vi "next chunk - read freq PID file.vi"(6 "temperature":dbl, 11 "peaks are known -- parameters":T1={"Gamma (kHz)"=0.0, "dV"=0.0, "time in Gamma (sec)"=0.0, "phi-star"=0.0, "all peaks exp (kHz)"=[564, 649, 987, 1133, 1214, 1585, 1763, 1823, 1880, 1899, 2032, 2138, 2221, 2270, 2350, 2456, 2580, 2634, 2831, 2960, 2965, 3131, 3328, 3469, 3553, 0, 3615, 3734, 0, 0, 0, 4236, 4300, 4331], "delta t (sec)"=0.0, "freq PID file path"=path "E:/data/Ultrasound/Experiment/ProbeTest/Probe10/YBCO_5/sweep4/9w/rus_scan_freq_list.dat", "default step (Hz)"=0.0}) -> (0 "temperatures":i32[](array[numeric]), 1 "frequencies":dbl[][](array[numeric]), 2 "PID freq":dbl[](array[numeric]))   [LabVIEW 2010]
uses:
  next chunk -- parameters.ctl
  <vilib>/Utility/file.llb/Read From Spreadsheet File (string).vi
panel:
  out "number 2":i32=9
  out "number":i32=9
  out "first line":string="Temperature(K)\tFrequency(kHz)\tGamma(kHz)\tDeltaFreq(kHz)\tTime(min)"
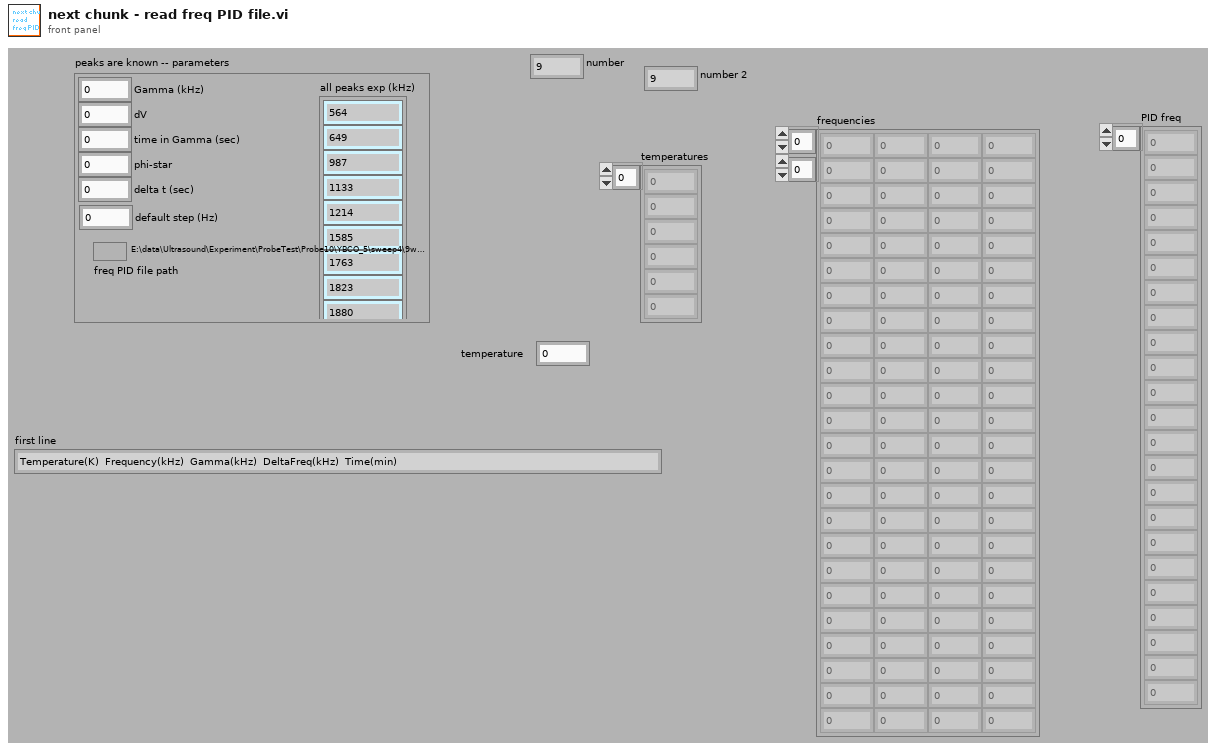
[diagram p1: front panel]
types:
  T1 = typedef "next chunk -- parameters.ctl" = cluster{"Gamma (kHz)":dbl, "dV":dbl, "time in Gamma (sec)":dbl, "phi-star":dbl, "all peaks exp (kHz)":i32[], "delta t (sec)":dbl, "freq PID file path":path, "default step (Hz)":dbl}
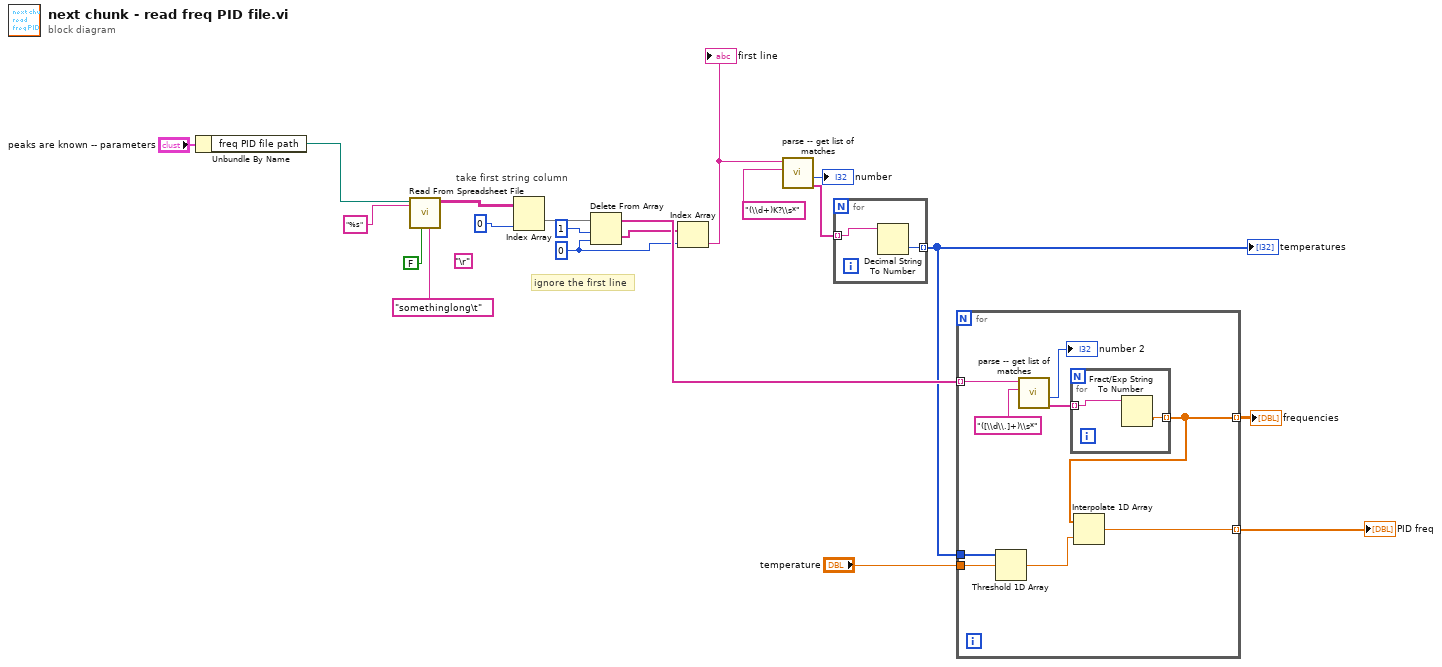
[diagram p0: block diagram]
diagram:
  w10 = 0 ("index")
  (unwired) "\r"
  # "take first string column"
  # "ignore the first line"
  n1 = Unbundle By Name("peaks are known -- parameters") -> ("freq PID file path"=w9:path)
  n2 = call-poly <vilib>:"Read From Spreadsheet File.vi"("delimiter (\\t)"="somethinglong\t" ("delimiter (\\t)"), "transpose (no:F)"=FALSE ("append to file? (new file:F)"), "format (%s)"="%s", "file path (dialog if empty)"=w9) -> ("all rows"=w16:string[][])  [unwired: 3 in, 4 out]
  n3 = Index Array(array=w16, index (col)=0 ("disabled index (col)")) -> (element=w14:string[])  [unwired: 1 in]
  n4 = Delete From Array(array=w14, length=1, index=w10) -> (deleted portion=w11:string[], array with subset deleted=w12:string[])
  n5 = Index Array(array=w11, index=w10) -> (element=w8:string)
  "first line" <- w8
  n6 = call "parse -- get list of matches.vi"("regexp"="(\\d+)K?\\s*", "string"=w8) -> ("Array"=w5:string[], "number of free elastic constants"=→"number":i32)  [unwired: 7 in, 1 out]
  n7 = for {
    tunnel: w5 -> [w22] mode=indexing
    tunnel: [w21] -> w3 mode=indexing
    n8 = Decimal String To Number(string=w22) -> (number=w21:i32)  [unwired: 2 in, 1 out]
  }
  "temperatures" <- w3
  n9 = for {
    tunnel: w12 -> [w29] mode=indexing
    tunnel: [w24] -> w4 mode=indexing
    tunnel: w3 -> [w27]
    tunnel: "temperature" -> [w26]
    tunnel: [w23] -> w1 mode=indexing
    n10 = Threshold 1D Array(2:w26, 3:w27) -> (0:w25:dbl)  [unwired: 1 in]
    n11 = call "parse -- get list of matches.vi"("regexp"="([\\d\\.]+)\\s*", "string"=w29) -> ("Array"=w30:string[], "number of free elastic constants"=→"number 2":i32)  [unwired: 7 in, 1 out]
    n12 = for {
      tunnel: w30 -> [w33] mode=indexing
      tunnel: [w32] -> w24 mode=indexing
      n13 = Fract/Exp String To Number(string=w33) -> (number=w32:dbl)  [unwired: 3 in, 1 out]
    }
    n14 = Interpolate 1D Array(1:w25, 2:w24) -> (0:w23:dbl)
  }
  "frequencies" <- w4
  "PID freq" <- w1
